vi "MenuSelect.vi"(8 "error in":errorcluster caption="错误输入（无错误）", 10 "Tag":string, 11 "PanelRootNode 输入":refnum<class "PanelRootNode.lvclass"> caption="DNL_LabVIEW Object in") -> (0 "error out":errorcluster caption="错误输出", 3 "PanelRootNode 输出":refnum<class "PanelRootNode.lvclass"> caption="DNL_LabVIEW Object out")   [LabVIEW 2013, in "PanelRootNode.lvclass"]
uses:
  PanelRootNode.lvclass
  PanelDataNode/Split Mode.ctl
  PanelDataNode/PanelDataNode.lvclass
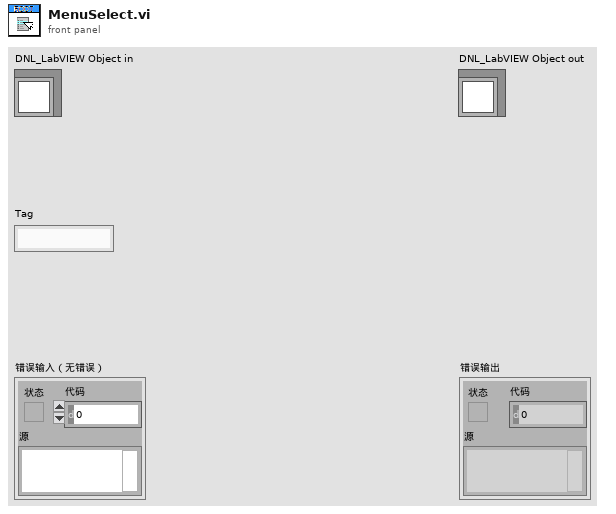
[diagram p1: front panel]
types:
  T1 = typedef "PanelDataNode.lvclass/Split Mode.ctl" = enum16{"Horizontal(up)", "Vertical(left)", "Horizontal(down)", "Vertical(right)"}
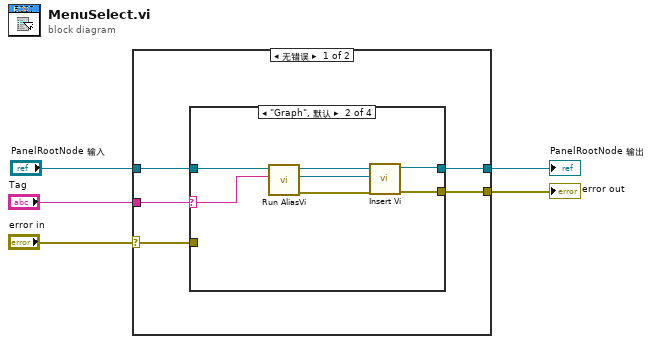
[diagram p0: block diagram]
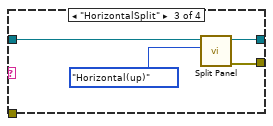
[diagram p3: hidden frame]
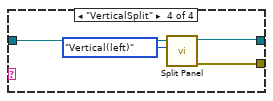
[diagram p4: hidden frame]
diagram:
  n1 = case shown="无错误" "error in" {
    selector: "error in" -> [w6 w29]
    tunnel: [w7 w29] -> w4
    tunnel: [w9 w28] -> w2
    tunnel: "PanelRootNode 输入" -> [w10 w28]
    tunnel: "Tag" -> [w8 _]
    frame No Error {
      n2 = case shown="\"Graph\", 默认" w8 {
        selector: w8 -> [_ w14 _ _]
        tunnel: w10 -> [w12 w19 w23 w27]
        tunnel: [w12 w17 w22 w26] -> w9
        tunnel: [w11 w13 w20 w24] -> w7
        tunnel: w6 -> [w11 _ _ _]
        frame "" {
        }
        frame "Graph", Default {
          n3 = call-dynamic "Run AliasVi.vi"("Vi Alias"=w14, "PanelDataNode 输入"=w19) -> ("error out"=w15:errorcluster, "VI*"=w16:refnum<vi>, "PanelDataNode 输出"=w18:refnum<class "PanelRootNode.lvclass">)  [unwired: 7 in]
          n4 = call-dynamic "Insert Vi.vi"("error in (no error)"=w15, "VI*"=w16, "PanelDataNode 输入"=w18) -> ("error out"=w13:errorcluster, "PanelDataNode 输出"=w17:refnum<class "PanelRootNode.lvclass">)  [unwired: 7 in]
        }
        frame "HorizontalSplit" {
          n5 = call-dynamic "Split Panel.vi"("Split Mode"=Split_Mode."Horizontal(up)", "PanelDataNode 输入"=w23) -> ("error out"=w20:errorcluster, "PanelDataNode 输出"=w22:refnum<class "PanelRootNode.lvclass">)  [unwired: 7 in, 1 out]
        }
        frame "VerticalSplit" {
          n6 = call-dynamic "Split Panel.vi"("Split Mode"=Split_Mode."Vertical(left)", "PanelDataNode 输入"=w27) -> ("error out"=w24:errorcluster, "PanelDataNode 输出"=w26:refnum<class "PanelRootNode.lvclass">)  [unwired: 7 in, 1 out]
        }
      }
    }
    frame Error {
    }
  }
  "error out" <- w4
  "PanelRootNode 输出" <- w2
